vi "Compile Protocol.vi"(8 "error in (no error)":errorcluster, 11 "Python Protocol in":refnum<class "Python Protocol.lvclass">) -> (0 "error out":errorcluster, 3 "Python Protocol out":refnum<class "Python Protocol.lvclass">)   [LabVIEW 2012, in "Python Protocol Actor.lvlib" / "Python Protocol.lvclass"]
uses:
  Python Protocol.lvclass
  Python Protocol.lvclass/Python Protocol.ctl
  Read Compiler.vi
  Read Code.vi
  Read Start Time.vi
  Read DVR.vi
  Read Refresh.vi
  <userlib>/_OpenG.lib/labpython/labpython.llb/PYTHON Set Float Data__ogtk.vi
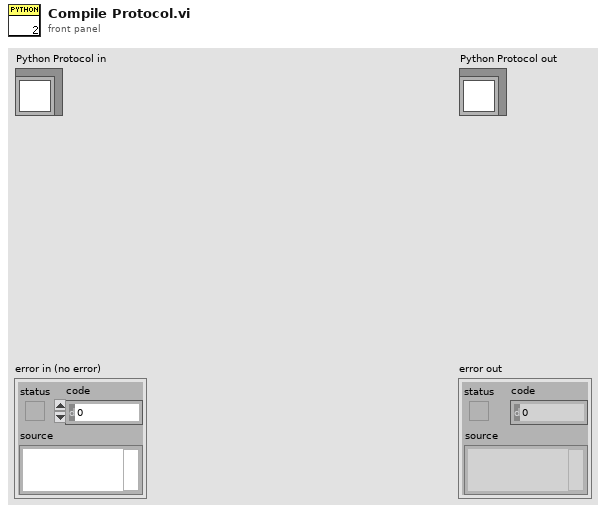
[diagram p1: front panel]
types:
  T1 = cluster{"Name":string, "Value":dbl, "Setpoint":dbl, "Output":dbl}[]
  T2 = typedef "PYTHON Session Refnum__ogtk.ctl" = refnum<k1>
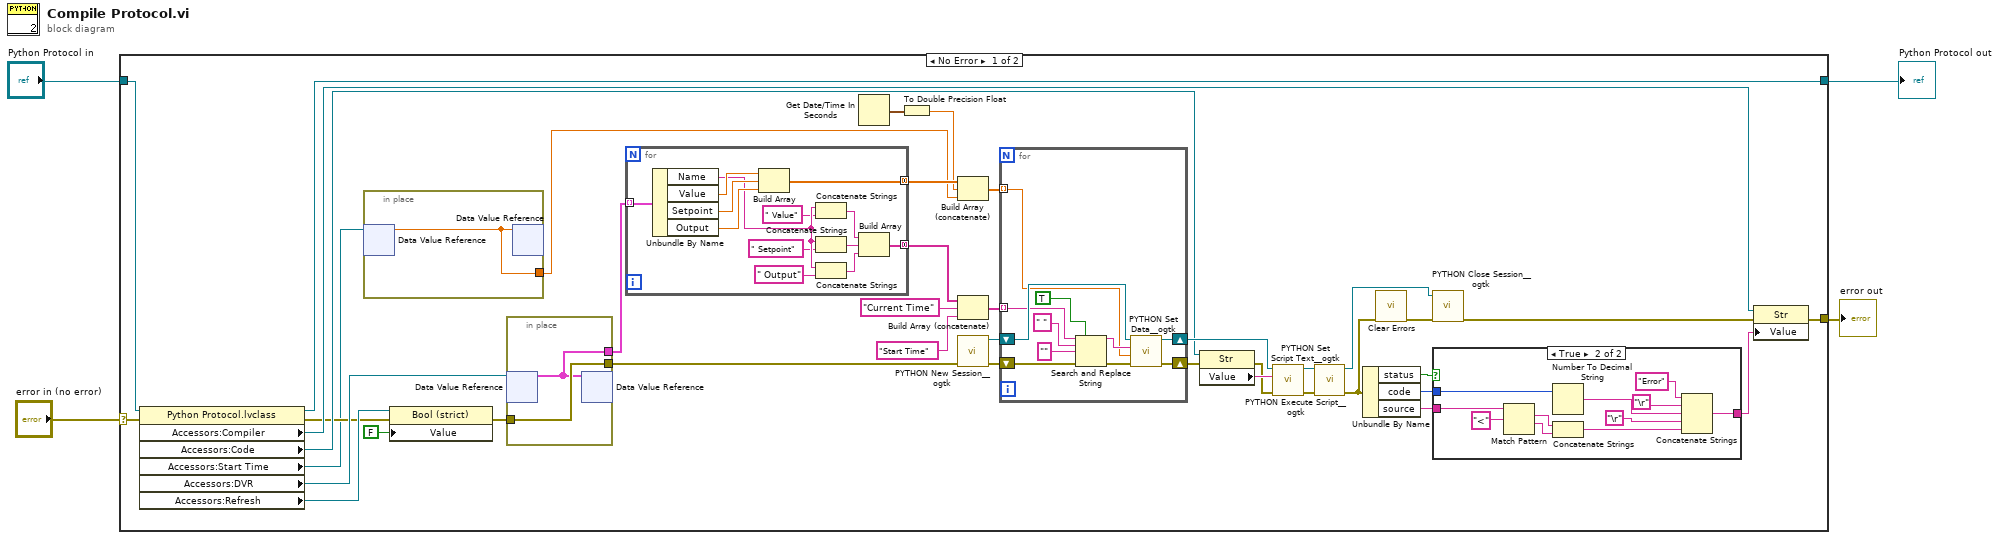
[diagram p0: block diagram]
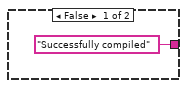
[diagram p2: hidden frame]
diagram:
  n1 = case shown="No Error" "error in (no error)" {
    selector: "error in (no error)" -> [w17 w84]
    tunnel: [w16 w84] -> w3
    tunnel: [w23 w83] -> w1
    tunnel: "Python Protocol in" -> [w24 w83]
    frame No Error {
      n2 = property class="Python Protocol.lvclass"(reference=w24, error in=w17) -> (reference out=w23:refnum<class "Python Protocol.lvclass">, error out=w18:errorcluster, "Accessors:Compiler"=w22:refnum<vi>, "Accessors:Code"=w21:refnum<vi>, "Accessors:Start Time"=w5:refnum<data-value>, "Accessors:DVR"=w20:refnum<data-value>, "Accessors:Refresh"=w19:refnum<vi>)
      n3 = in-place {
        in-place-border: [w44] -> w6
        n4 = in-place-dvr #1(w5) -> (w44:dbl)  [unwired: 1 out]
        n5 = in-place-dvr #1(w44) -> ()  [unwired: 2 out]
      }
      n6 = property class="Bool (strict)"(reference=w19, error in=w18, "Value"=FALSE) -> (error out=w26:errorcluster)  [unwired: 1 out]
      n7 = in-place {
        in-place-border: [w82] -> w27
        in-place-border: w26 -> [w82]
        in-place-border: [w81] -> w14
        n8 = in-place-dvr #2(w20) -> (w81:T1)  [unwired: 1 out]
        n9 = in-place-dvr #2(w81) -> ()  [unwired: 2 out]
      }
      n10 = for {
        tunnel: w14 -> [w57] mode=indexing
        tunnel: [w46] -> w9 mode=concatenating
        tunnel: [w45] -> w13 mode=concatenating
        n11 = Unbundle By Name(w57) -> ("Name"=w53:string, "Value"=w54:dbl, "Setpoint"=w55:dbl, "Output"=w56:dbl)
        n12 = Build Array(w54, w55, w56) -> (w45:dbl[])
        n13 = Concatenate Strings(w53, " Value" ("string")) -> (w49:string)
        n14 = Concatenate Strings(w53, " Setpoint" ("string")) -> (w48:string)
        n15 = Concatenate Strings(w53, " Output" ("string")) -> (w47:string)
        n16 = Build Array(w49, w48, w47) -> (w46:string[])
      }
      n17 = Get Date/Time In Seconds() -> (seconds since 1Jan1904=w15:timestamp)
      n18 = To Double Precision Float(number=w15) -> (double precision float=w7:dbl)
      n19 = Build Array (concatenate)(w13, w7, w6) -> (w12:dbl[])
      n20 = Build Array (concatenate)(w9, "Current Time", "Start Time" ("element")) -> (w8:string[])
      n21 = call <userlib>:"PYTHON New Session__ogtk.vi"("error in (no error)"=w27) -> ("error out"=w40:errorcluster, "Python Session"=w39:T2)  [unwired: 5 in]
      n22 = for {
        tunnel: w8 -> [w75] mode=indexing
        shift-right: [w79] -> w41
        shift-left: w39 -> [w78]
        shift-right: [w80] -> w36
        shift-left: w40 -> [w77]
        tunnel: w12 -> [w70] mode=indexing
        n23 = Search and Replace String(replace all?=TRUE ("replace all? (F)"), input string=w75, search string=" ", replace string="" ("replace string (\"\")"), error in=w77) -> (result string=w71:string, error out=w76:errorcluster)  [unwired: 3 in, 2 out]
        n24 = call-poly <userlib>:"PYTHON Set Data__ogtk.vi"("error in (no error)"=w76, "value"=w70, "variable name"=w71, "Python Session in"=w78) -> ("error out"=w80:errorcluster, "Python Session out"=w79:T2)  [unwired: 2 in]
      }
      n25 = property class="Str"(reference=w21, error in=w36) -> (error out=w37:errorcluster, "Value"=w38:string)  [unwired: 1 out]
      n26 = call <userlib>:"PYTHON Set Script Text__ogtk.vi"("error in (no error)"=w37, "script text"=w38, "Python Session in"=w41) -> ("error out"=w42:errorcluster, "Python Session out"=w43:T2)  [unwired: 3 in]
      n27 = call <userlib>:"PYTHON Execute Script__ogtk.vi"("error in (no error)"=w42, "Python Session in"=w43) -> ("error out"=w28:errorcluster, "Python Session out"=w30:T2)  [unwired: 4 in]
      n28 = Unbundle By Name(w28) -> ("status"=w33:bool, "code"=w35:i32, "source"=w34:string)
      n29 = call <vilib>:"Clear Errors.vi"("error in (no error)"=w28) -> ("error out"=w31:errorcluster)  [unwired: 6 in]
      n30 = call <userlib>:"PYTHON Close Session__ogtk.vi"("error in (no error)"=w31, "Python Session in"=w30) -> ("error out"=w29:errorcluster)  [unwired: 5 in]
      n31 = case shown="True" w33 {
        tunnel: w35 -> [_ w69]
        tunnel: w34 -> [_ w63]
        tunnel: ["Successfully compiled" w66] -> w32
        frame False {
        }
        frame True {
          n32 = Match Pattern(string=w63, regular expression="<") -> (match substring=w61:string, after substring=w60:string)  [unwired: 1 in, 2 out]
          n33 = Number To Decimal String(number=w69) -> (decimal integer string=w68:string)  [unwired: 1 in]
          n34 = Concatenate Strings(w61, w60) -> (w59:string)
          n35 = Concatenate Strings("Error" ("string"), "\r", w68, "\r", w59) -> (w66:string)
        }
      }
      n36 = property class="Str"(reference=w22, error in=w29, "Value"=w32) -> (error out=w16:errorcluster)  [unwired: 1 out]
    }
    frame Error {
    }
  }
  "error out" <- w3
  "Python Protocol out" <- w1
